vi "Configure Autozero.vi"(8 "error in (no error)":errorcluster, 10 "Enable Autozero (True)":bool=TRUE, 11 "VISA resource name":refnum<visa-resource-name>) -> (0 "error out":errorcluster, 3 "VISA resource name out":refnum<visa-resource-name>)   [LabVIEW 2015, in "Voltech PM1000+.lvlib"]
doc: "Enables or disables the autozero function on the instrument. Enabling autozero optimizes the instrument for accuracy, while disabling optimizes for speed.\n\nNormally the PM1000+ will cancel any small dc offsets in the measurement automatically. This is called Auto Zero. Auto Zero should always be enabled."
uses:
  <instrlib>/Voltech PM1000+/Voltech PM1000+.lvlib
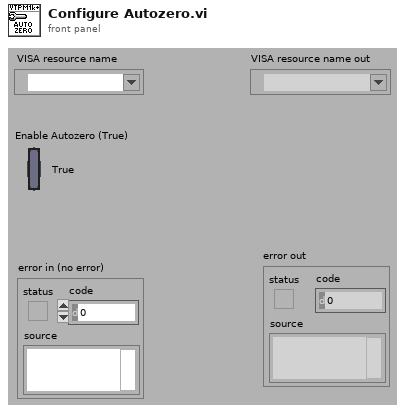
[diagram p1: front panel]
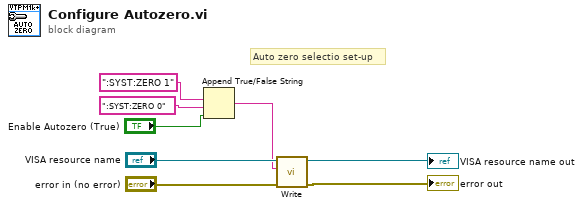
[diagram p0: block diagram]
diagram:
  # "Auto zero selectio set-up"
  n1 = Append True/False String(1:"Enable Autozero (True)", 2:":SYST:ZERO 0" ("Disable Autozero"), 3:":SYST:ZERO 1" ("Enable Autozero")) -> (0:w3:string)  [unwired: 1 in]
  n2 = call <instrlib>:"Write.vi"("error in (no error)"="error in (no error)", "Write Buffer"=w3, "VISA resource name"="VISA resource name") -> ("error out"=→"error out":errorcluster, "VISA resource name out"=→"VISA resource name out":refnum<visa-resource-name>)  [unwired: 7 in]
